vi "add all digests.vi"(8 "error in":errorcluster, 11 "force?":bool) -> (0 "error out":errorcluster)   [LabVIEW 2016, in "lvlibcrypto digest.lvclass"]
uses:
  lvlibcrypto digest.lvclass
  lv tls dll.lvlib
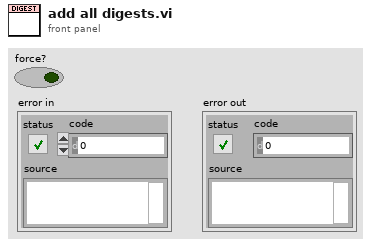
[diagram p1: front panel]
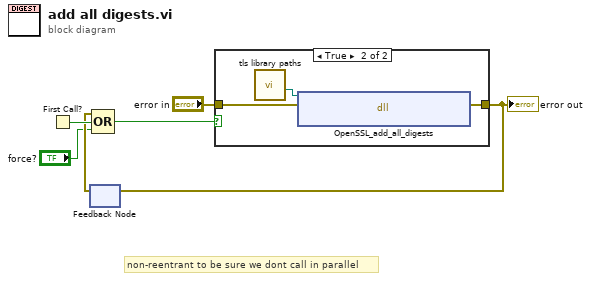
[diagram p0: block diagram]
diagram:
  # "non-reentrant to be sure we dont call in parallel"
  n1 = First Call?() -> (First Call?: T/F=w5:bool)
  n2 = feedback #1() -> (w4:errorcluster)  [unwired: 1 in]
  n3 = Compound Arithmetic op=OR(w4, w5, "force?") -> (w2:bool)
  n4 = case shown="True" w2 {
    tunnel: "error in" -> [w7 w10]
    tunnel: [w7 w8] -> w3
    frame False {
    }
    frame True {
      n5 = call "tls library paths.vi"() -> ("libcrypto"=w9:path)  [unwired: 8 in, 3 out]
      n6 = dll-call lib="C:/Users/IEUser/Desktop/tlssimple/libcrypto-41.dll" fn="OpenSSL_add_all_digests"(path in=w9, error in=w10) -> (error out=w8:errorcluster)  [unwired: 2 in, 1 out]
    }
  }
  "error out" <- w3
  n7 = feedback-in #1(w3) -> ()
